vi "CommonVIs_EvaluateMethodText.vi"(1 "String":string) -> (13 "MethodAttributeName":string, 14 "Protected":bool, 16 "MethodName":string, 17 "Private":bool, 18 "MethodType":string, 19 "SetMethod":bool)   [LabVIEW 2020]
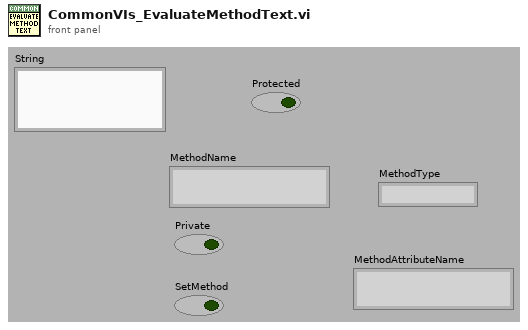
[diagram p1: front panel]
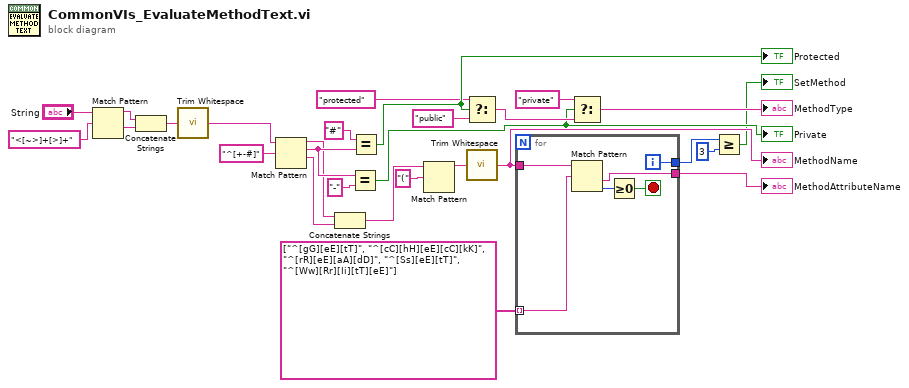
[diagram p0: block diagram]
diagram:
  n1 = Match Pattern(string="String", regular expression="<[~>]+[>]+") -> (before substring=w13:string, after substring=w14:string)  [unwired: 3 out]
  n2 = Concatenate Strings(w13, w14) -> (w12:string)
  n3 = call <vilib>:"Trim Whitespace.vi"("string"=w12) -> ("trimmed string"=w24:string)  [unwired: 1 in]
  n4 = Match Pattern(string=w24, regular expression="^[+-#]") -> (before substring=w18:string, match substring=w27:string, after substring=w19:string)  [unwired: 2 out]
  n5 = Concatenate Strings(w18, w19) -> (w22:string)
  n6 = Equal?(x=w27, y="-") -> (x = y?=w9:bool)
  "Private" <- w9
  n7 = Equal?(x="#", y=w27) -> (x = y?=w8:bool)
  "Protected" <- w8
  n8 = Match Pattern(string=w22, regular expression="(") -> (before substring=w25:string)  [unwired: 4 out]
  n9 = Select(t="protected", s=w8, f="public") -> (s? t:f=w10:string)
  n10 = call <vilib>:"Trim Whitespace.vi"("string"=w25) -> ("trimmed string"=w26:string)  [unwired: 1 in]
  "MethodName" <- w26
  n11 = for {
    tunnel: w26 -> [w33]
    tunnel: string[] ["^[gG][eE][tT]", "^[cC][hH][eE][cC][kK]", "^[rR][eE][aA][dD]", "^[Ss][eE][tT]", "^[Ww][Rr][Ii][tT][eE]"] -> [w32] mode=indexing
    tunnel: [w30] -> w4
    tunnel: [w29] -> w1
    i -> [w30]
    stop <- w31 stop-if-true
    n12 = Match Pattern(string=w33, regular expression=w32) -> (after substring=w29:string, offset past match=w34:i32)  [unwired: 3 out]
    n13 = Greater Or Equal To 0?(x=w34) -> (x >= 0?=w31:bool)
  }
  "MethodAttributeName" <- w1
  n14 = Select(t="private", s=w9, f=w10) -> (s? t:f=→"MethodType":string)
  n15 = Greater Or Equal?(x=w4, y=3) -> (x >= y?=→"SetMethod":bool)
